vi "matching_numbers.vi"() -> ()   [LabVIEW 2025]
uses:
  <vilib>/numeric/Random Number (Range) I64.vi
  <vilib>/numeric/sub_Random U32.vi
panel:
  out "iteration 0-1":i32
  out "iteration 0-1000":i32
  out "number":dbl
  out "Waveform Graph 2":i32[](graph)
  out "random number":i64
  out "Waveform Graph":i64[](graph)
  in  "number sleected by the user":i16=80 min=0 max=1000 step=1
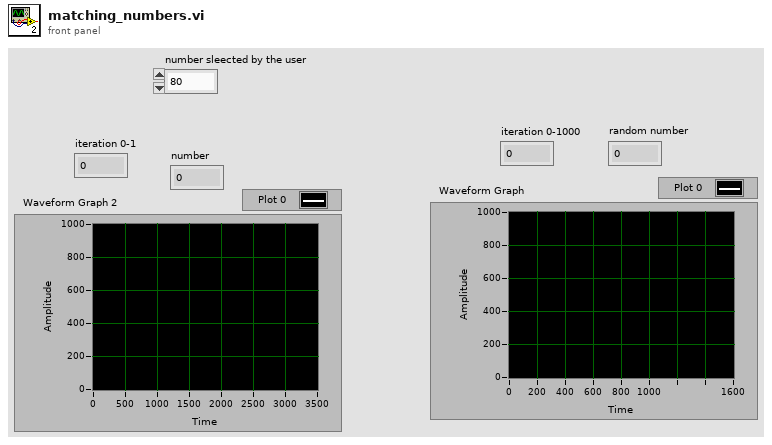
[diagram p1: front panel]
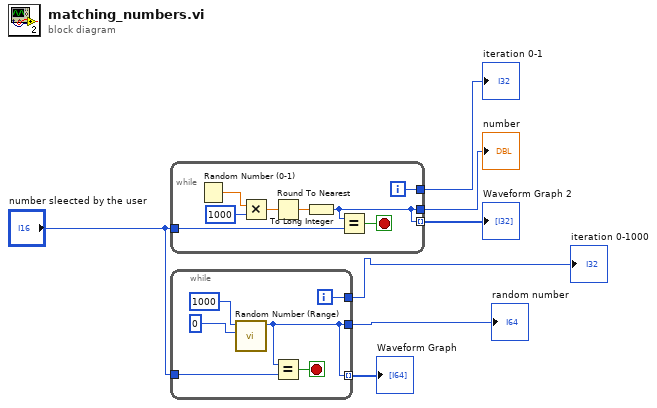
[diagram p0: block diagram]
diagram:
  n1 = while {
    tunnel: "number sleected by the user" -> [w12]
    tunnel: [w8] -> w4 mode=indexing
    tunnel: [w8] -> w3
    tunnel: [w11] -> w1
    i -> [w11]
    stop <- w13 stop-if-true
    n2 = Random Number (0-1)() -> (number: 0 to 1=w15:dbl)
    n3 = Multiply(x=w15, y=i16 1000) -> (x*y=w10:dbl)
    n4 = Round To Nearest(number=w10) -> (nearest integer value=w9:dbl)
    n5 = To Long Integer(number=w9) -> (32bit integer=w8:i32)
    n6 = Equal?(x=w8, y=w12) -> (x = y?=w13:bool)
  }
  "Waveform Graph 2" <- w4
  "number" <- w3
  "iteration 0-1" <- w1
  n7 = while {
    tunnel: "number sleected by the user" -> [w20]
    tunnel: [w17] -> w7 mode=indexing
    tunnel: [w17] -> w6
    tunnel: [w16] -> w2
    i -> [w16]
    stop <- w21 stop-if-true
    n8 = call-poly <vilib>:"Random Number (Range).vi"("lower bound (-100)"=i64 0, "upper bound (100)"=i64 1000) -> ("number"=w17:i64)  [unwired: 9 in]
    n9 = Equal?(x=w17, y=w20) -> (x = y?=w21:bool)
  }
  "Waveform Graph" <- w7
  "random number" <- w6
  "iteration 0-1000" <- w2
